vi "closeSEDSpect.vi"(8 "error in (no error)":errorcluster, 11 "Model in":refnum<class "Model.lvclass">) -> (0 "error out":errorcluster, 3 "Model out":refnum<class "Model.lvclass">)   [LabVIEW 2016, in "Model.lvclass"]
uses:
  Model.lvclass
  Model.lvclass/Model.ctl
  ss_sedspectrometer/SEDSpectrometer/SEDSpectrometer.lvclass
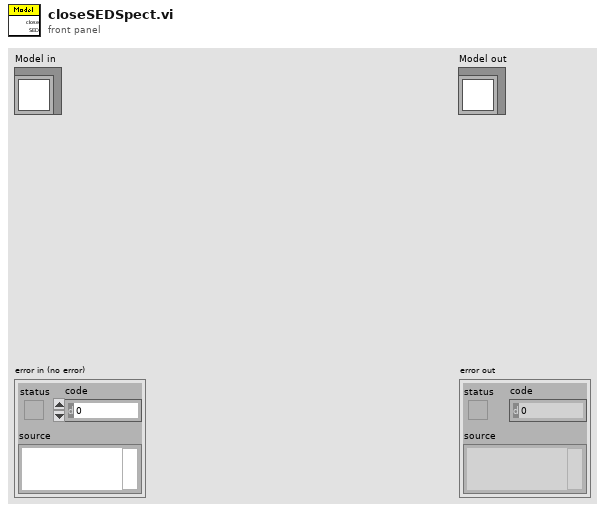
[diagram p1: front panel]
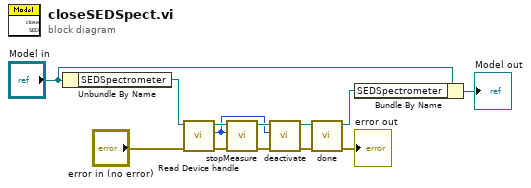
[diagram p0: block diagram]
diagram:
  n1 = Unbundle By Name("Model in") -> ("SEDSpectrometer"=w3:refnum<class "SEDSpectrometer.lvclass">)
  n2 = call-dynamic "Read Device handle.vi"("error in (no error)"="error in (no error)", "SEDSpectrometer in"=w3) -> ("error out"=w10:errorcluster, "Device handle"=w7:i32, "SEDSpectrometer out"=w9:refnum<class "SEDSpectrometer.lvclass">)  [unwired: 7 in]
  n3 = call "stopMeasure.vi"("error in (no error)"=w10, "Device"=w7, "SEDSpectrometer in"=w9) -> ("error out"=w11:errorcluster, "SEDSpectrometer out"=w8:refnum<class "SEDSpectrometer.lvclass">)  [unwired: 6 in, 1 out]
  n4 = call "deactivate.vi"("error in (no error)"=w11, "Handle"=w7, "SEDSpectrometer in"=w8) -> ("error out"=w12:errorcluster, "SEDSpectrometer out"=w13:refnum<class "SEDSpectrometer.lvclass">)  [unwired: 6 in, 1 out]
  n5 = call "done.vi"("error in (no error)"=w12, "SEDSpectrometer in"=w13) -> ("error out"=→"error out":errorcluster, "SEDSpectrometer out"=w4:refnum<class "SEDSpectrometer.lvclass">)  [unwired: 7 in, 1 out]
  n6 = Bundle By Name(cluster="Model in", "SEDSpectrometer"=w4) -> (→"Model out":refnum<class "Model.lvclass">)
